vi "Write Label Props.vi"(8 "error in (no error)":errorcluster, 10 "Label Props":T1, 11 "Ctl Refnum in":refnum<vi>) -> (0 "error out":errorcluster, 3 "Ctl Refnum":refnum<vi>)   [LabVIEW 2020, in "VolatusGUIEditorCore.lvlib"]
uses:
  VolatusGUIEditorCore.lvlib
  Label Props.ctl
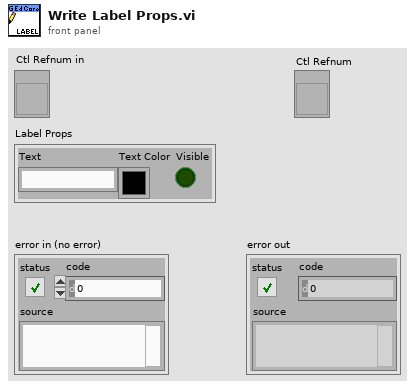
[diagram p1: front panel]
types:
  T1 = typedef "VolatusGUIEditorCore.lvlib/Label Props.ctl" = cluster{"Text":string, "Text Color":u32, "Visible":bool}
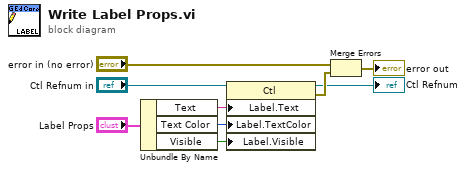
[diagram p0: block diagram]
diagram:
  n1 = Unbundle By Name("Label Props") -> ("Text"=w6:string, "Text Color"=w7:u32, "Visible"=w5:bool)
  n2 = property class="Ctl"(reference="Ctl Refnum in", "Label.Text"=w6, "Label.TextColor"=w7, "Label.Visible"=w5) -> (reference out=→"Ctl Refnum":refnum<vi>, error out=w3:errorcluster)  [unwired: 1 in]
  n3 = Merge Errors("error in (no error)", w3) -> (→"error out":errorcluster)
